vi "Prompt for Step.vi"(8 "error in (no error)":errorcluster, 10 "Subpanel Ref":refnum<vi>, 11 "Timing Action in":refnum<class "Timing Action.lvclass">) -> (0 "error out":errorcluster, 3 "Timing Action out":refnum<class "Timing Action.lvclass">)   [LabVIEW 2020, in "MacroAssert.lvlib" / "Timing Action.lvclass"]
doc: "Displays its own window into <B>Subpanel Ref</B> for the user to enter a macro step."
uses:
  Timing Action.lvclass
  Action Step/Action Step.lvclass
panel:
  in  "Time to Wait Until":timestamp format="%<%.3X>T"
  in  "Time to Wait":dbl min=0.0
  in  "Time Unit":u16(ring) items=["milliseconds", "seconds", "minutes"]
  out "Subtype Description":string
  in  "Step Subtype":u16(ring) items=["Wait", "Wait Until"]
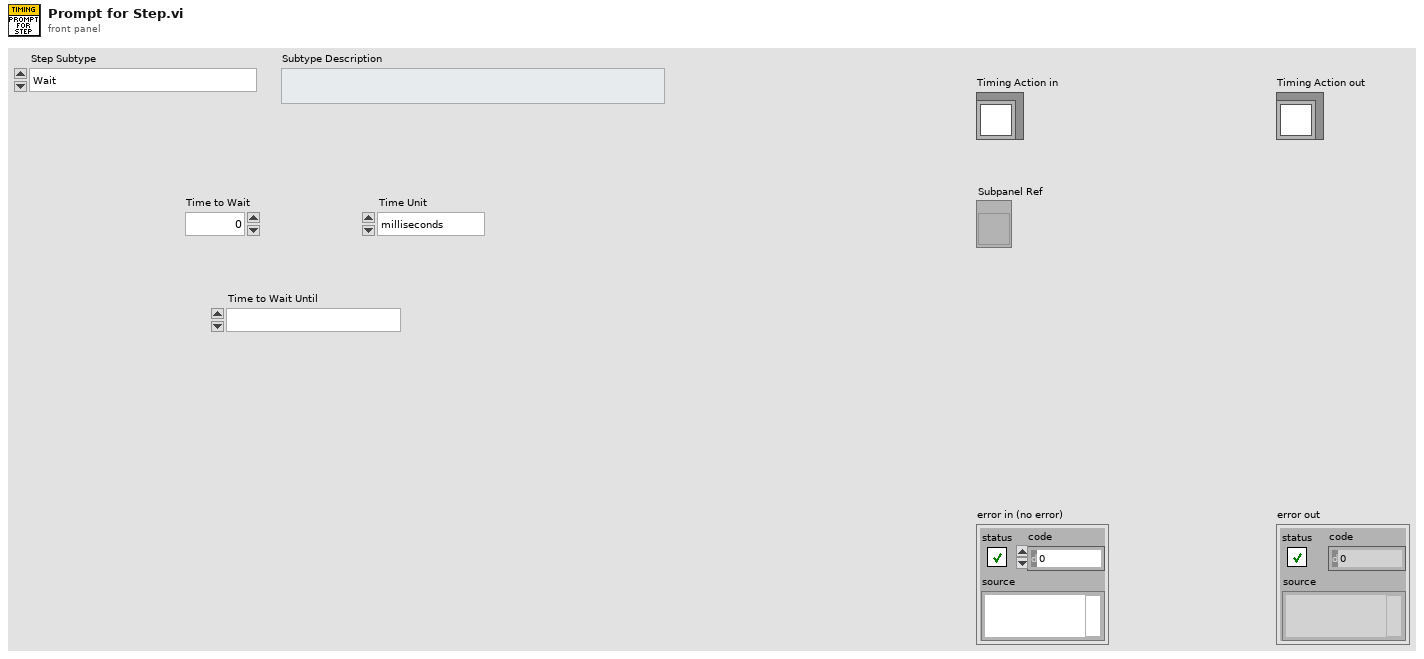
[diagram p1: front panel]
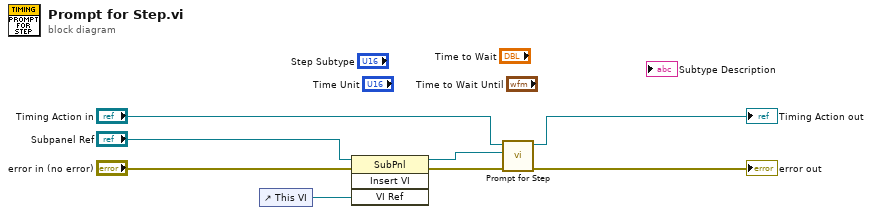
[diagram p0: block diagram]
diagram:
  n1 = control-ref of="This VI"() -> (w6:refnum<vi>)
  n2 = invoke class="SubPnl" method="Insert VI"(reference="Subpanel Ref", error in="error in (no error)", "VI Ref"=w6) -> (reference out=w7:refnum<vi>, error out=w8:errorcluster)  [unwired: 1 in, 2 out]
  n3 = call-parent "Prompt for Step.vi"("error in (no error)"=w8, "Subpanel Ref"=w7, "Step in"="Timing Action in") -> ("error out"=→"error out":errorcluster, "Step out"=→"Timing Action out":refnum<class "Timing Action.lvclass">)  [unwired: 7 in]
